vi "CH4.vi"() -> ()   [LabVIEW 2021]
panel:
  in  "CH4":cluster{"CH4 Array":dbl[], "CH4 Message":string}
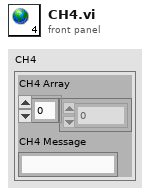
[diagram p1: front panel]
diagram:
